vi "GetListener.vi"(1 "TestResult in":refnum<class "TestResult.lvclass">) -> (0 "Listener":refnum<class "TestListener.lvclass">)   [LabVIEW 2017, in "TestResult.lvclass"]
doc: "Returns the listener."
uses:
  TestResult.lvclass
  TestListener/TestListener.lvclass
  TestResult.lvclass/TestResult.ctl
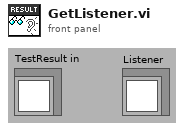
[diagram p1: front panel]
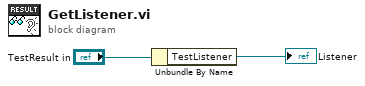
[diagram p0: block diagram]
diagram:
  n1 = Unbundle By Name("TestResult in") -> ("TestListener"=→"Listener":refnum<class "TestListener.lvclass">)
